vi "Error.vi"(1 "Popup?":bool=TRUE, 2 "Error String":string, 3 "Error In":bool) -> (0 "Error":bool)   [LabVIEW 2014]
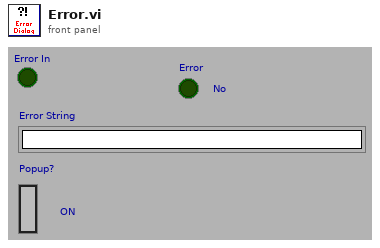
[diagram p1: front panel]
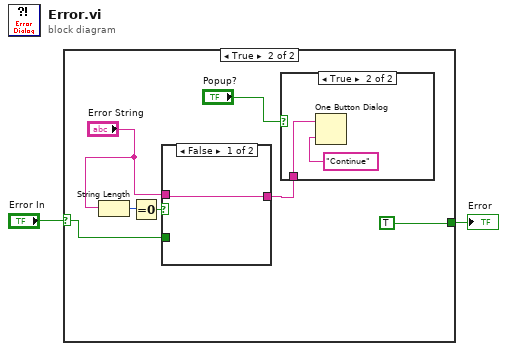
[diagram p0: block diagram]
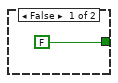
[diagram p2: hidden frame]
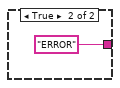
[diagram p4: hidden frame]
diagram:
  n1 = case shown="True" "Error In" {
    selector: "Error In" -> [_ w7]
    tunnel: [FALSE TRUE] -> w1
    frame False {
    }
    frame True {
      n2 = String Length(string="Error String") -> (length=w8:i32)
      n3 = Equal To 0?(x=w8) -> (x = 0?=w9:bool)
      n4 = case shown="False" w9 {
        tunnel: [w13 "ERROR"] -> w5
        tunnel: "Error String" -> [w13 _]
        tunnel: w7 -> [_ _]
        frame False {
        }
        frame True {
        }
      }
      n5 = case shown="True" "Popup?" {
        tunnel: w5 -> [_ w11]
        frame False {
        }
        frame True {
          n6 = One Button Dialog(message=w11, button name ("OK")="Continue") -> ()  [unwired: 1 out]
        }
      }
    }
  }
  "Error" <- w1
